vi "putty.vi"(10 "makeTimestamp":bool) -> ()   [LabVIEW 2011, in "run.lvlib"]
uses:
  run.lvlib
  Tools/Filing.lvlib
  Tools/Filing/FileNeologist/FileNeologist.lvclass
panel:
  out "standard error 2":string
  out "standard output 2":string
  out "Network Drive path (local)":path
  out "standard error":string
  out "standard output":string
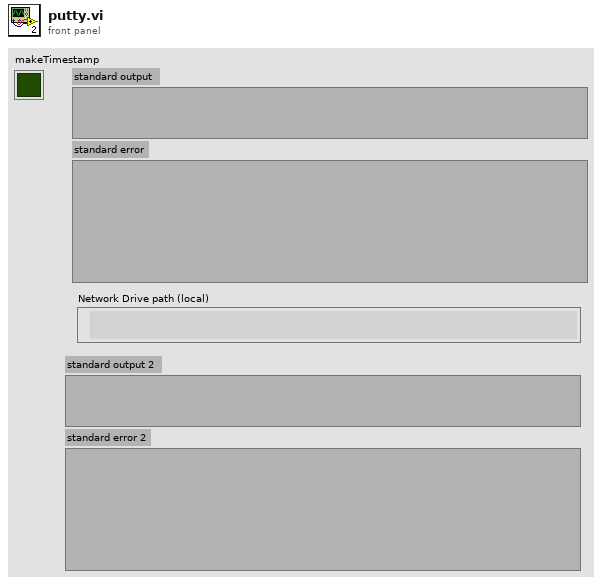
[diagram p1: front panel]
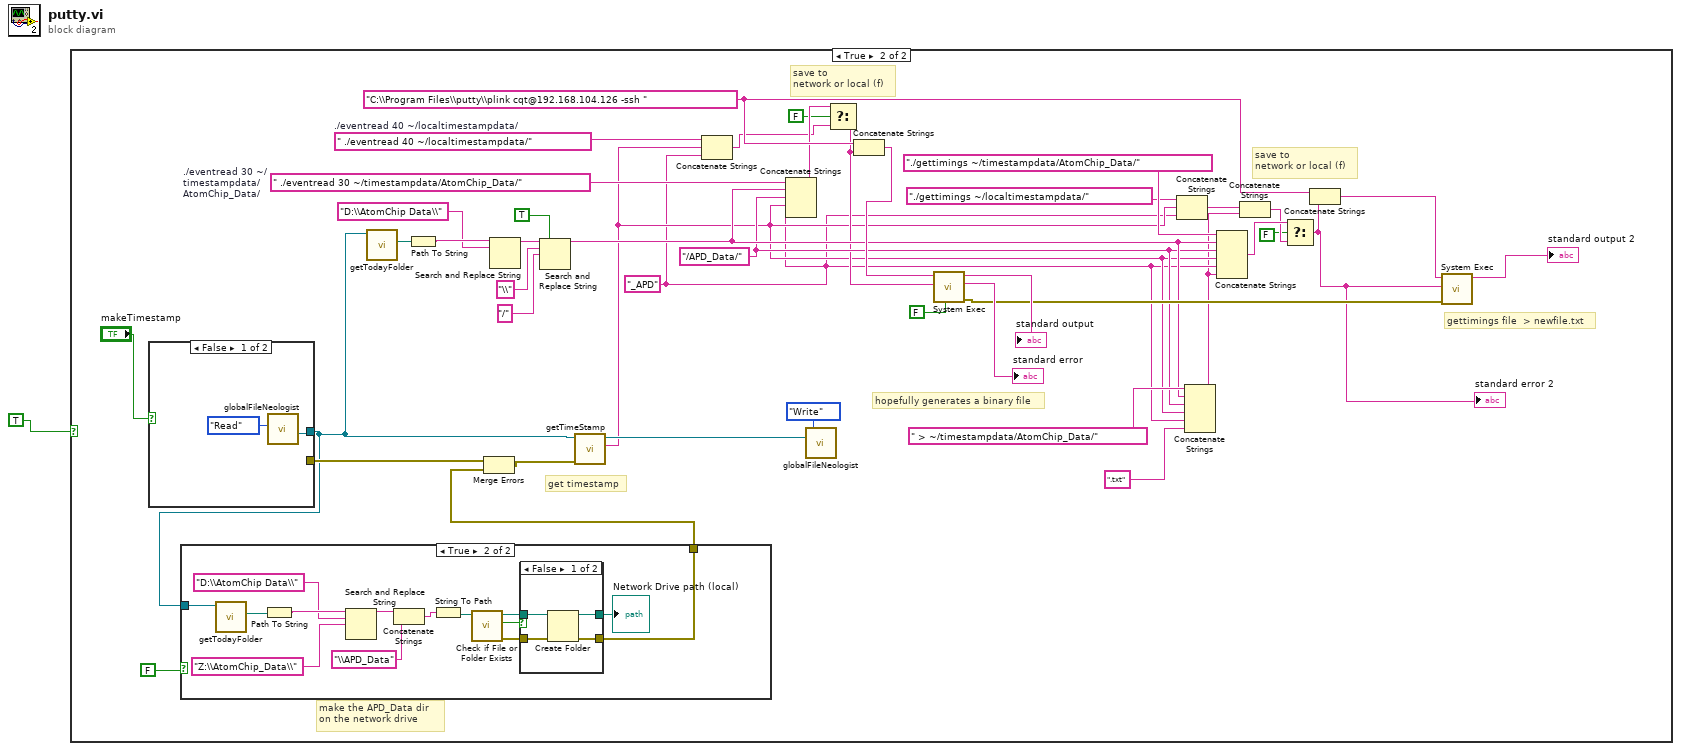
[diagram p0: block diagram]
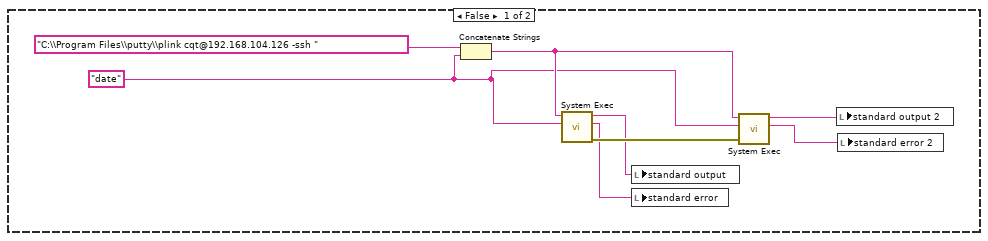
[diagram p2: hidden frame]
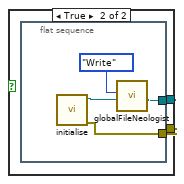
[diagram p5: hidden frame]
diagram:
  n1 = case shown="True" TRUE {
    frame False {
      w6 = "date"
      n2 = Concatenate Strings("C:\\Program Files\\putty\\plink cqt@192.168.104.126 -ssh " ("command line"), w6) -> (w7:string)
      n3 = call <vilib>:"System Exec.vi"("standard input"=w6, "command line"=w7) -> ("error out"=w8:errorcluster, "standard error"=w4:string, "standard output"=w5:string)  [unwired: 6 in, 1 out]
      n4 = local write "standard output"(w5) -> ()
      n5 = local write "standard error"(w4) -> ()
      n6 = call <vilib>:"System Exec.vi"("error in (no error)"=w8, "standard input"=w6, "command line"=w7) -> ("standard error"=w2:string, "standard output"=w3:string)  [unwired: 5 in, 2 out]
      n7 = local write "standard output 2"(w3) -> ()
      n8 = local write "standard error 2"(w2) -> ()
    }
    frame True {
      w24 = " ./eventread 40 ~/localtimestampdata/"  # ./eventread 40 ~/localtimestampdata/
      w27 = "/APD_Data/"
      w51 = " ./eventread 30 ~/timestampdata/AtomChip_Data/"  # ./eventread 30 ~/timestampdata/AtomChip_Data/
      w17 = "_APD"
      w34 = "C:\\Program Files\\putty\\plink cqt@192.168.104.126 -ssh " ("command line")
      # "save to\nnetwork or local (f)"
      # "save to\nnetwork or local (f)"
      # "hopefully generates a binary file"
      # "gettimings file  > newfile.txt"
      # "make the APD_Data dir \non the network drive"
      # "get timestamp"
      n9 = case shown="False" "makeTimestamp" {
        tunnel: [_ w76] -> w43
        tunnel: [w73 w75] -> w40
        frame False {
          n10 = call "globalFileNeologist.vi"("Action"=enum16{"Write", "Read"}."Read") -> ("FileNeologist out"=w73:refnum<class "FileNeologist.lvclass">)  [unwired: 10 in]
        }
        frame True {
          n11 = flat-sequence {
            tunnel: [w80] -> w76
            tunnel: [w77] -> w75
            frame #0 {
              n12 = call "initialise.vi"() -> ("error out"=w80:errorcluster, "FileNeologist out"=w78:refnum<class "FileNeologist.lvclass">)  [unwired: 10 in]
              n13 = call "globalFileNeologist.vi"("FileNeologist in"=w78, "Action"=enum16{"Write", "Read"}."Write") -> ("FileNeologist out"=w77:refnum<class "FileNeologist.lvclass">)  [unwired: 9 in]
            }
          }
        }
      }
      n14 = case shown="True" FALSE {
        tunnel: [_ w54] -> w42
        tunnel: w40 -> [_ w53]
        frame False {
        }
        frame True {
          n15 = call "getTodayFolder.vi"("FileNeologist in"=w53) -> ("todayFolder"=w66:path)  [unwired: 8 in, 2 out]
          n16 = Path To String(path=w66) -> (string=w65:string)
          n17 = Search and Replace String(input string=w65, search string="D:\\AtomChip Data\\" ("search string/char (-)"), replace string="Z:\\AtomChip_Data\\" ("search string/char (-)")) -> (result string=w59:string)  [unwired: 5 in, 3 out]
          n18 = Concatenate Strings(w59, "\\APD_Data" ("search string/char (-)")) -> (w56:string)
          n19 = String To Path(string=w56) -> (path=w57:path)
          n20 = call <vilib>:"Check if File or Folder Exists.vi"("path"=w57) -> ("error out"=w60:errorcluster, "file or folder exists?"=w62:bool, "dup path"=w61:path)  [unwired: 8 in]
          n21 = case shown="False" w62 {
            tunnel: w61 -> [w70 w72]
            tunnel: [w67 w72] -> w55
            tunnel: w60 -> [w69 w71]
            tunnel: [w68 w71] -> w54
            frame False {
              n22 = Create Folder(path (use dialog)=w70, error in=w69) -> (created path=w67:path, error out=w68:errorcluster)  [unwired: 1 in, 1 out]
            }
            frame True {
            }
          }
          "Network Drive path (local)" <- w55
        }
      }
      n23 = call "getTodayFolder.vi"("FileNeologist in"=w40) -> ("todayFolder"=w46:path)  [unwired: 8 in, 2 out]
      n24 = Path To String(path=w46) -> (string=w45:string)
      n25 = Merge Errors(w43, w42) -> (w41:errorcluster)
      n26 = Search and Replace String(input string=w45, search string="D:\\AtomChip Data\\" ("search string/char (-)")) -> (result string=w39:string)  [unwired: 6 in, 3 out]
      n27 = Search and Replace String(replace all?=TRUE ("replace all? (F)"), input string=w39, search string="\\", replace string="/") -> (result string=w28:string)  [unwired: 4 in, 3 out]
      n28 = call "getTimeStamp.vi"("error in (no error)"=w41, "FileNeologist in"=w40) -> ("TimeStamp"=w18:string, "FileNeologist out"=w48:refnum<class "FileNeologist.lvclass">)  [unwired: 7 in, 1 out]
      n29 = Concatenate Strings(w24, w18, w17) -> (w22:string)
      n30 = Concatenate Strings(w51, w28, w27, w18, w17) -> (w23:string)
      n31 = call "globalFileNeologist.vi"("FileNeologist in"=w48, "Action"=enum16{"Write", "Read"}."Write") -> ()  [unwired: 9 in, 1 out]
      n32 = Select(t=w23, s=FALSE ("Boolean"), f=w22) -> (s? t:f=w21:string)
      n33 = Concatenate Strings(w34, w21) -> (w50:string)
      n34 = call <vilib>:"System Exec.vi"("run minimized? (F)"=FALSE, "standard input"=w21, "command line"=w50) -> ("error out"=w30:errorcluster, "standard error"=→"standard error":string, "standard output"=→"standard output":string)  [unwired: 5 in, 1 out]
      n35 = Concatenate Strings("./gettimings ~/localtimestampdata/", w18, w17) -> (w16:string)
      n36 = Concatenate Strings(" > ~/timestampdata/AtomChip_Data/", w28, w27, w18, w17, ".txt") -> (w15:string)
      n37 = Concatenate Strings("./gettimings ~/timestampdata/AtomChip_Data/", w28, w27, w18, w17, w15) -> (w14:string)
      n38 = Concatenate Strings(w16, w15) -> (w13:string)
      n39 = Select(t=w14, s=FALSE ("Boolean"), f=w13) -> (s? t:f=w12:string)
      "standard error 2" <- w12
      n40 = Concatenate Strings(w34, w12) -> (w33:string)
      n41 = call <vilib>:"System Exec.vi"("error in (no error)"=w30, "standard input"=w12, "command line"=w33) -> ("standard output"=→"standard output 2":string)  [unwired: 5 in, 3 out]
    }
  }
